vi "GeoData.vi"() -> ()   [LabVIEW 2017] (continued)
TX\tDallas County\tH1\n75007\t48113\tCarrollton\tTX\tDallas County\tH1\n76065\t48113\tMidlothian\tTX\tDallas County\tH1\n75376\t48113\tDallas\tTX\tDallas County\tH1\n75382\t48113\tDallas\tTX\tDallas County\tH1\n75015\t48113\tIrving\tTX\tDallas County\tH1\n75185\t48113\tMesquite\tTX\tDallas County\tH1\n75260\t48113\tDallas\tTX\tDallas County\tH1\n75030\t48113\tRowlett\tTX\tDallas County\tH1\n75125\t48113\tFerris\tTX\tDallas County\tH1\n75206\t48113\tDallas\tTX\tDallas County\tH1\n75229\t48113\tDallas\tTX\tDallas County\tH1\n75218\t48113\tDallas\tTX\tDallas County\tH1\n75248\t48113\tDallas\tTX\tDallas County\tH1\n75054\t48113\tGrand prairie\tTX\tDallas County\tH1\n75082\t48113\tRichardson\tTX\tDallas County\tH1\n75182\t48113\tSunnyvale\tTX\tDallas County\tH1\n75380\t48113\tDallas\tTX\tDallas County\tH1\n75313\t48113\tDallas\tTX\tDallas County\tH1\n75367\t48113\tDallas\tTX\tDallas County\tH1\n75038\t48113\tIrving\tTX\tDallas County\tH1\n75042\t48113\tGarland\tTX\tDallas County\tH1\n75052\t48113\tGrand prairie\tTX\tDallas County\tH1\n75104\t48113\tCedar hill\tTX\tDallas County\tH1\n75150\t48113\tMesquite\tTX\tDallas County\tH1\n75207\t48113\tDallas\tTX\tDallas County\tH1\n75154\t48113\tRed oak\tTX\tDallas County\tH1\n75209\t48113\tDallas\tTX\tDallas County\tH1\n75219\t48113\tDallas\tTX\tDallas County\tH1\n75222\t48113\tDallas\tTX\tDallas County\tH1\n75063\t48113\tIrving\tTX\tDallas County\tH1\n75083\t48113\tRichardson\tTX\tDallas County\tH1\n75081\t48113\tRichardson\tTX\tDallas County\tH1\n75270\t48113\tDallas\tTX\tDallas County\tH1\n75381\t48113\tDallas\tTX\tDallas County\tH1\n75017\t48113\tIrving\tTX\tDallas County\tH1\n75372\t48113\tDallas\tTX\tDallas County\tH1\n79713\t48115\tAckerly\tTX\tDawson County\tH1\n79331\t48115\tLamesa\tTX\tDawson County\tH1\n79377\t48115\tWelch\tTX\tDawson County\tH1\n79351\t48115\tOdonnell\tTX\tDawson County\tH1\n79045\t48117\tHereford\tTX\tDeaf Smith County\tH1\n79098\t48117\tWildorado\tTX\tDeaf Smith County\tH1\n79025\t48117\tDawn\tTX\tDeaf Smith County\tH1\n79092\t48117\tVega\tTX\tDeaf Smith County\tH1\n79035\t48117\tFriona\tTX\tDeaf Smith County\tH1\n79085\t48117\tSummerfield\tTX\tDeaf Smith County\tH1\n79015\t48117\tCanyon\tTX\tDeaf Smith County\tH1\n75469\t48119\tPecan gap\tTX\tDelta County\tH1\n75432\t48119\tCooper\tTX\tDelta County\tH1\n75428\t48119\tCommerce\tTX\tDelta County\tH1\n75450\t48119\tLake creek\tTX\tDelta County\tH1\n75415\t48119\tBen franklin\tTX\tDelta County\tH1\n75448\t48119\tKlondike\tTX\tDelta County\tH1\n75449\t48119\tLadonia\tTX\tDelta County\tH1\n75441\t48119\tEnloe\tTX\tDelta County\tH1\n75067\t48121\tLewisville\tTX\tDenton County\tH1\n76207\t48121\tDenton\tTX\tDenton County\tH1\n76259\t48121\tPonder\tTX\tDenton County\tH1\n76202\t48121\tDenton\tTX\tDenton County\tH1\n76078\t48121\tRhome\tTX\tDenton County\tH1\n76262\t48121\tRoanoke\tTX\tDenton County\tH1\n76258\t48121\tPilot point\tTX\tDenton County\tH1\n75029\t48121\tLewisville\tTX\tDenton County\tH1\n76206\t48121\tDenton\tTX\tDenton County\tH1\n75033\t48121\tFrisco\tTX\tDenton County\tH1\n75077\t48121\tLewisville\tTX\tDenton County\tH1\n75010\t48121\tCarrollton\tTX\tDenton County\tH1\n76205\t48121\tDenton\tTX\tDenton County\tH1\n76210\t48121\tDenton\tTX\tDenton County\tH1\n76177\t48121\tFort worth\tTX\tDenton County\tH1\n76204\t48121\tDenton\tTX\tDenton County\tH1\n75019\t48121\tCoppell\tTX\tDenton County\tH1\n75287\t48121\tDallas\tTX\tDenton County\tH1\n76092\t48121\tSouthlake\tTX\tDenton County\tH1\n76234\t48121\tDecatur\tTX\tDenton County\tH1\n76247\t48121\tJustin\tTX\tDenton County\tH1\n75065\t48121\tLake dallas\tTX\tDenton County\tH1\n75009\t48121\tCelina\tTX\tDenton County\tH1\n76208\t48121\tDenton\tTX\tDenton County\tH1\n76226\t48121\tArgyle\tTX\tDenton County\tH1\n75011\t48121\tCarrollton\tTX\tDenton County\tH1\n75028\t48121\tFlower mound\tTX\tDenton County\tH1\n75093\t48121\tPlano\tTX\tDenton County\tH1\n75007\t48121\tCarrollton\tTX\tDenton County\tH1\n76249\t48121\tKrum\tTX\tDenton County\tH1\n76201\t48121\tDenton\tTX\tDenton County\tH1\n76266\t48121\tSanger\tTX\tDenton County\tH1\n75027\t48121\tFlower mound\tTX\tDenton County\tH1\n75022\t48121\tFlower mound\tTX\tDenton County\tH1\n75024\t48121\tPlano\tTX\tDenton County\tH1\n75057\t48121\tLewisville\tTX\tDenton County\tH1\n76052\t48121\tHaslet\tTX\tDenton County\tH1\n76209\t48121\tDenton\tTX\tDenton County\tH1\n76203\t48121\tDenton\tTX\tDenton County\tH1\n75034\t48121\tFrisco\tTX\tDenton County\tH1\n75035\t48121\tFrisco\tTX\tDenton County\tH1\n75068\t48121\tLittle elm\tTX\tDenton County\tH1\n75056\t48121\tThe colony\tTX\tDenton County\tH1\n75078\t48121\tProsper\tTX\tDenton County\tH1\n76227\t48121\tAubrey\tTX\tDenton County\tH1\n76272\t48121\tValley view\tTX\tDenton County\tH1\n77967\t48123\tHochheim\tTX\tDeWitt County\tH1\n77954\t48123\tCuero\tTX\tDeWitt County\tH1\n77984\t48123\tShiner\tTX\tDeWitt County\tH1\n77974\t48123\tMeyersville\tTX\tDeWitt County\tH1\n78141\t48123\tNordheim\tTX\tDeWitt County\tH1\n77989\t48123\tThomaston\tTX\tDeWitt County\tH1\n77995\t48123\tYoakum\tTX\tDeWitt County\tH1\n77994\t48123\tWesthoff\tTX\tDeWitt County\tH1\n78164\t48123\tYorktown\tTX\tDeWitt County\tH1\n79256\t48125\tRoaring springs\tTX\tDickens County\tH1\n79370\t48125\tSpur\tTX\tDickens County\tH1\n79220\t48125\tAfton\tTX\tDickens County\tH1\n79229\t48125\tDickens\tTX\tDickens County\tH1\n79243\t48125\tMcadoo\tTX\tDickens County\tH1\n78827\t48127\tAsherton\tTX\tDimmit County\tH1\n78836\t48127\tCatarina\tTX\tDimmit County\tH1\n78834\t48127\tCarrizo springs\tTX\tDimmit County\tH1\n78839\t48127\tCrystal city\tTX\tDimmit County\tH1\n78830\t48127\tBig wells\tTX\tDimmit County\tH1\n79065\t48129\tPampa\tTX\tDonley County\tH1\n79237\t48129\tHedley\tTX\tDonley County\tH1\n79057\t48129\tMclean\tTX\tDonley County\tH1\n79226\t48129\tClarendon\tTX\tDonley County\tH1\n79240\t48129\tLelia lake\tTX\tDonley County\tH1\n78357\t48131\tFreer\tTX\tDuval County\tH1\n78384\t48131\tSan diego\tTX\tDuval County\tH1\n78332\t48131\tAlice\tTX\tDuval County\tH1\n78349\t48131\tConcepcion\tTX\tDuval County\tH1\n78376\t48131\tRealitos\tTX\tDuval County\tH1\n78341\t48131\tBenavides\tTX\tDuval County\tH1\n76435\t48133\tCarbon\tTX\tEastland County\tH1\n76470\t48133\tRanger\tTX\tEastland County\tH1\n76471\t48133\tRising star\tTX\tEastland County\tH1\n76466\t48133\tOlden\tTX\tEastland County\tH1\n76442\t48133\tComanche\tTX\tEastland County\tH1\n76444\t48133\tDe leon\tTX\tEastland County\tH1\n76437\t48133\tCisco\tTX\tEastland County\tH1\n76464\t48133\tMoran\tTX\tEastland County\tH1\n76445\t48133\tDesdemona\tTX\tEastland County\tH1\n76443\t48133\tCross plains\tTX\tEastland County\tH1\n76448\t48133\tEastland\tTX\tEastland County\tH1\n76454\t48133\tGorman\tTX\tEastland County\tH1\n79760\t48135\tOdessa\tTX\tEctor County\tH1\n79762\t48135\tOdessa\tTX\tEctor County\tH1\n79707\t48135\tMidland\tTX\tEctor County\tH1\n79763\t48135\tOdessa\tTX\tEctor County\tH1\n79765\t48135\tOdessa\tTX\tEctor County\tH1\n79768\t48135\tOdessa\tTX\tEctor County\tH1\n79741\t48135\tGoldsmith\tTX\tEctor County\tH1\n79761\t48135\tOdessa\tTX\tEctor County\tH1\n79764\t48135\tOdessa\tTX\tEctor County\tH1\n79758\t48135\tGardendale\tTX\tEctor County\tH1\n79766\t48135\tOdessa\tTX\tEctor County\tH1\n79776\t48135\tPenwell\tTX\tEctor County\tH1\n79769\t48135\tOdessa\tTX\tEctor County\tH1\n79759\t48135\tNotrees\tTX\tEctor County\tH1\n78833\t48137\tCamp wood\tTX\tEdwards County\tH1\n78880\t48137\tRocksprings\tTX\tEdwards County\tH1\n78840\t48137\tDel rio\tTX\tEdwards County\tH1\n78828\t48137\tBarksdale\tTX\tEdwards County\tH1\n75146\t48139\tLancaster\tTX\tEllis County\tH1\n76055\t48139\tItasca\tTX\tEllis County\tH1\n75152\t48139\tPalmer\tTX\tEllis County\tH1\n76084\t48139\tVenus\tTX\tEllis County\tH1\n76041\t48139\tForreston\tTX\tEllis County\tH1\n75165\t48139\tWaxahachie\tTX\tEllis County\tH1\n76641\t48139\tFrost\tTX\tEllis County\tH1\n76651\t48139\tItaly\tTX\tEllis County\tH1\n76626\t48139\tBlooming grove\tTX\tEllis County\tH1\n75119\t48139\tEnnis\tTX\tEllis County\tH1\n75167\t48139\tWaxahachie\tTX\tEllis County\tH1\n76050\t48139\tGrandview\tTX\tEllis County\tH1\n76064\t48139\tMaypearl\tTX\tEllis County\tH1\n76065\t48139\tMidlothian\tTX\tEllis County\tH1\n75168\t48139\tWaxahachie\tTX\tEllis County\tH1\n75125\t48139\tFerris\tTX\tEllis County\tH1\n76063\t48139\tMansfield\tTX\tEllis County\tH1\n76670\t48139\tMilford\tTX\tEllis County\tH1\n75104\t48139\tCedar hill\tTX\tEllis County\tH1\n75154\t48139\tRed oak\tTX\tEllis County\tH1\n76623\t48139\tAvalon\tTX\tEllis County\tH1\n75101\t48139\tBardwell\tTX\tEllis County\tH1\n79836\t48141\tClint\tTX\tEl Paso County\tH1\n79923\t48141\tEl paso\tTX\tEl Paso County\tH1\n79932\t48141\tEl paso\tTX\tEl Paso County\tH1\n79936\t48141\tEl paso\tTX\tEl Paso County\tH1\n79931\t48141\tEl paso\tTX\tEl Paso County\tH1\n79948\t48141\tEl paso\tTX\tEl Paso County\tH1\n79953\t48141\tEl paso\tTX\tEl Paso County\tH1\n79905\t48141\tEl paso\tTX\tEl Paso County\tH1\n79914\t48141\tEl paso\tTX\tEl Paso County\tH1\n79927\t48141\tEl paso\tTX\tEl Paso County\tH1\n79911\t48141\tEl paso\tTX\tEl Paso County\tH1\n79937\t48141\tEl paso\tTX\tEl Paso County\tH1\n79910\t48141\tEl paso\tTX\tEl Paso County\tH1\n79912\t48141\tEl paso\tTX\tEl Paso County\tH1\n79915\t48141\tEl paso\tTX\tEl Paso County\tH1\n79930\t48141\tEl paso\tTX\tEl Paso County\tH1\n79926\t48141\tEl paso\tTX\tEl Paso County\tH1\n79944\t48141\tEl paso\tTX\tEl Paso County\tH1\n79935\t48141\tEl paso\tTX\tEl Paso County\tH1\n79996\t48141\tEl paso\tTX\tEl Paso County\tH1\n79942\t48141\tEl paso\tTX\tEl Paso County\tH1\n79968\t48141\tEl paso\tTX\tEl Paso County\tH1\n79954\t48141\tEl paso\tTX\tEl Paso County\tH1\n79835\t48141\tCanutillo\tTX\tEl Paso County\tH1\n79902\t48141\tEl paso\tTX\tEl Paso County\tH1\n79907\t48141\tEl paso\tTX\tEl Paso County\tH1\n79849\t48141\tSan elizario\tTX\tEl Paso County\tH1\n79903\t48141\tEl paso\tTX\tEl Paso County\tH1\n79908\t48141\tEl paso\tTX\tEl Paso County\tH1\n79941\t48141\tEl paso\tTX\tEl Paso County\tH1\n79951\t48141\tEl paso\tTX\tEl Paso County\tH1\n79952\t48141\tEl paso\tTX\tEl Paso County\tH1\n79940\t48141\tEl paso\tTX\tEl Paso County\tH1\n79924\t48141\tEl paso\tTX\tEl Paso County\tH1\n79904\t48141\tEl paso\tTX\tEl Paso County\tH1\n79906\t48141\tEl paso\tTX\tEl Paso County\tH1\n79938\t48141\tEl paso\tTX\tEl Paso County\tH1\n79934\t48141\tEl paso\tTX\tEl Paso County\tH1\n79821\t48141\tAnthony\tTX\tEl Paso County\tH1\n79913\t48141\tEl paso\tTX\tEl Paso County\tH1\n79955\t48141\tEl paso\tTX\tEl Paso County\tH1\n79838\t48141\tFabens\tTX\tEl Paso County\tH1\n79946\t48141\tEl paso\tTX\tEl Paso County\tH1\n79901\t48141\tEl paso\tTX\tEl Paso County\tH1\n79922\t48141\tEl paso\tTX\tEl Paso County\tH1\n79928\t48141\tEl paso\tTX\tEl Paso County\tH1\n79997\t48141\tEl paso\tTX\tEl Paso County\tH1\n79950\t48141\tEl paso\tTX\tEl Paso County\tH1\n79995\t48141\tEl paso\tTX\tEl Paso County\tH1\n79945\t48141\tEl paso\tTX\tEl Paso County\tH1\n79918\t48141\tFort bliss\tTX\tEl Paso County\tH1\n79925\t48141\tEl paso\tTX\tEl Paso County\tH1\n79943\t48141\tEl paso\tTX\tEl Paso County\tH1\n79917\t48141\tEl paso\tTX\tEl Paso County\tH1\n79916\t48141\tFort bliss\tTX\tEl Paso County\tH1\n79929\t48141\tEl paso\tTX\tEl Paso County\tH1\n79947\t48141\tEl paso\tTX\tEl Paso County\tH1\n79853\t48141\tTornillo\tTX\tEl Paso County\tH1\n79949\t48141\tEl paso\tTX\tEl Paso County\tH1\n76436\t48143\tCarlton\tTX\tErath County\tH1\n76462\t48143\tLipan\tTX\tErath County\tH1\n76401\t48143\tStephenville\tTX\tErath County\tH1\n76453\t48143\tGordon\tTX\tErath County\tH1\n76461\t48143\tLingleville\tTX\tErath County\tH1\n76446\t48143\tDublin\tTX\tErath County\tH1\n76457\t48143\tHico\tTX\tErath County\tH1\n76433\t48143\tBluff dale\tTX\tErath County\tH1\n76649\t48143\tIredell\tTX\tErath County\tH1\n76465\t48143\tMorgan mill\tTX\tErath County\tH1\n76444\t48143\tDe leon\tTX\tErath County\tH1\n76445\t48143\tDesdemona\tTX\tErath County\tH1\n76463\t48143\tMingus\tTX\tErath County\tH1\n76402\t48143\tStephenville\tTX\tErath County\tH1\n76629\t48145\tBremond\tTX\tFalls County\tH1\n76664\t48145\tMart\tTX\tFalls County\tH1\n76519\t48145\tBurlington\tTX\tFalls County\tH1\n76579\t48145\tTroy\tTX\tFalls County\tH1\n76655\t48145\tLorena\tTX\tFalls County\tH1\n76632\t48145\tChilton\tTX\tFalls County\tH1\n76630\t48145\tBruceville\tTX\tFalls County\tH1\n76682\t48145\tRiesel\tTX\tFalls County\tH1\n76570\t48145\tRosebud\tTX\tFalls County\tH1\n76706\t48145\tWaco\tTX\tFalls County\tH1\n76653\t48145\tKosse\tTX\tFalls County\tH1\n76680\t48145\tReagan\tTX\tFalls County\tH1\n76524\t48145\tEddy\tTX\tFalls County\tH1\n76661\t48145\tMarlin\tTX\tFalls County\tH1\n76685\t48145\tSatin\tTX\tFalls County\tH1\n76656\t48145\tLott\tTX\tFalls County\tH1\n75414\t48147\tBells\tTX\tFannin County\tH1\n75469\t48147\tPecan gap\tTX\tFannin County\tH1\n75438\t48147\tDodd city\tTX\tFannin County\tH1\n75423\t48147\tCeleste\tTX\tFannin County\tH1\n75447\t48147\tIvanhoe\tTX\tFannin County\tH1\n75418\t48147\tBonham\tTX\tFannin County\tH1\n75479\t48147\tSavoy\tTX\tFannin County\tH1\n75439\t48147\tEctor\tTX\tFannin County\tH1\n75476\t48147\tRavenna\tTX\tFannin County\tH1\n75475\t48147\tRandolph\tTX\tFannin County\tH1\n75496\t48147\tWolfe city\tTX\tFannin County\tH1\n75443\t48147\tGober\tTX\tFannin County\tH1\n75452\t48147\tLeonard\tTX\tFannin County\tH1\n75490\t48147\tTrenton\tTX\tFannin County\tH1\n75488\t48147\tTelephone\tTX\tFannin County\tH1\n75449\t48147\tLadonia\tTX\tFannin County\tH1\n75413\t48147\tBailey\tTX\tFannin County\tH1\n75424\t48147\tBlue ridge\tTX\tFannin County\tH1\n75446\t48147\tHoney grove\tTX\tFannin County\tH1\n75491\t48147\tWhitewright\tTX\tFannin County\tH1\n75492\t48147\tWindom\tTX\tFannin County\tH1\n78942\t48149\tGiddings\tTX\tFayette County\tH1\n78932\t48149\tCarmine\tTX\tFayette County\tH1\n78934\t48149\tColumbus\tTX\tFayette County\tH1\n78959\t48149\tWaelder\tTX\tFayette County\tH1\n78952\t48149\tPlum\tTX\tFayette County\tH1\n78949\t48149\tMuldoon\tTX\tFayette County\tH1\n78951\t48149\tOakland\tTX\tFayette County\tH1\n78941\t48149\tFlatonia\tTX\tFayette County\tH1\n78940\t48149\tFayetteville\tTX\tFayette County\tH1\n78956\t48149\tSchulenburg\tTX\tFayette County\tH1\n78946\t48149\tLedbetter\tTX\tFayette County\tH1\n78935\t48149\tAlleyton\tTX\tFayette County\tH1\n78954\t48149\tRound top\tTX\tFayette County\tH1\n78957\t48149\tSmithville\tTX\tFayette County\tH1\n78962\t48149\tWeimar\tTX\tFayette County\tH1\n78961\t48149\tWarrenton\tTX\tFayette County\tH1\n78960\t48149\tWarda\tTX\tFayette County\tH1\n78963\t48149\tWest point\tTX\tFayette County\tH1\n78950\t48149\tNew ulm\tTX\tFayette County\tH1\n78938\t48149\tEllinger\tTX\tFayette County\tH1\n78945\t48149\tLa grange\tTX\tFayette County\tH1\n79526\t48151\tHermleigh\tTX\tFisher County\tH1\n79520\t48151\tHamlin\tTX\tFisher County\tH1\n79545\t48151\tRoscoe\tTX\tFisher County\tH1\n79534\t48151\tMc caulley\tTX\tFisher County\tH1\n79543\t48151\tRoby\tTX\tFisher County\tH1\n79546\t48151\tRotan\tTX\tFisher County\tH1\n79560\t48151\tSylvester\tTX\tFisher County\tH1\n79556\t48151\tSweetwater\tTX\tFisher County\tH1\n79231\t48153\tDougherty\tTX\tFloyd County\tH1\n79241\t48153\tLockney\tTX\tFloyd County\tH1\n79235\t48153\tFloydada\tTX\tFloyd County\tH1\n79258\t48153\tSouth plains\tTX\tFloyd County\tH1\n79221\t48153\tAiken\tTX\tFloyd County\tH1\n79227\t48155\tCrowell\tTX\tFoard County\tH1\n76384\t48155\tVernon\tTX\tFoard County\tH1\n79248\t48155\tPaducah\tTX\tFoard County\tH1\n77469\t48157\tRichmond\tTX\tFort Bend County\tH1\n77489\t48157\tMissouri city\tTX\tFort Bend County\tH1\n77584\t48157\tPearland\tTX\tFort Bend County\tH1\n77476\t48157\tSimonton\tTX\tFort Bend County\tH1\n77417\t48157\tBeasley\tTX\tFort Bend County\tH1\n77031\t48157\tHouston\tTX\tFort Bend County\tH1\n77461\t48157\tNeedville\tTX\tFort Bend County\tH1\n77082\t48157\tHouston\tTX\tFort Bend County\tH1\n77407\t48157\tRichmond\tTX\tFort Bend County\tH1\n77441\t48157\tFulshear\tTX\tFort Bend County\tH1\n77471\t48157\tRosenberg\tTX\tFort Bend County\tH1\n77493\t48157\tKaty\tTX\tFort Bend County\tH1\n77487\t48157\tSugar land\tTX\tFort Bend County\tH1\n77497\t48157\tStafford\tTX\tFort Bend County\tH1\n77085\t48157\tHouston\tTX\tFort Bend County\tH1\n77423\t48157\tBrookshire\tTX\tFort Bend County\tH1\n77435\t48157\tEast bernard\tTX\tFort Bend County\tH1\n77420\t48157\tBoling\tTX\tFort Bend County\tH1\n77478\t48157\tSugar land\tTX\tFort Bend County\tH1\n77496\t48157\tSugar land\tTX\tFort Bend County\tH1\n77451\t48157\tKendleton\tTX\tFort Bend County\tH1\n77406\t48157\tRichmond\tTX\tFort Bend County\tH1\n77450\t48157\tKaty\tTX\tFort Bend County\tH1\n77498\t48157\tSugar land\tTX\tFort Bend County\tH1\n77583\t48157\tRosharon\tTX\tFort Bend County\tH1\n77464\t48157\tOrchard\tTX\tFort Bend County\tH1\n77430\t48157\tDamon\tTX\tFort Bend County\tH1\n77459\t48157\tMissouri city\tTX\tFort Bend County\tH1\n77444\t48157\tGuy\tTX\tFort Bend County\tH1\n77083\t48157\tHouston\tTX\tFort Bend County\tH1\n77053\t48157\tHouston\tTX\tFort Bend County\tH1\n77479\t48157\tSugar land\tTX\tFort Bend County\tH1\n77545\t48157\tFresno\tTX\tFort Bend County\tH1\n77481\t48157\tThompsons\tTX\tFort Bend County\tH1\n77099\t48157\tHouston\tTX\tFort Bend County\tH1\n77485\t48157\tWallis\tTX\tFort Bend County\tH1\n77494\t48157\tKaty\tTX\tFort Bend County\tH1\n77477\t48157\tStafford\tTX\tFort Bend County\tH1\n75457\t48159\tMount vernon\tTX\tFranklin County\tH1\n75480\t48159\tScroggins\tTX\tFranklin County\tH1\n75455\t48159\tMount pleasant\tTX\tFranklin County\tH1\n75481\t48159\tSulphur bluff\tTX\tFranklin County\tH1\n75494\t48159\tWinnsboro\tTX\tFranklin County\tH1\n75487\t48159\tTalco\tTX\tFranklin County\tH1\n75478\t48159\tSaltillo\tTX\tFranklin County\tH1\n75838\t48161\tDonie\tTX\tFreestone County\tH1\n75859\t48161\tStreetman\tTX\tFreestone County\tH1\n75840\t48161\tFairfield\tTX\tFreestone County\tH1\n76667\t48161\tMexia\tTX\tFreestone County\tH1\n75831\t48161\tBuffalo\tTX\tFreestone County\tH1\n75855\t48161\tOakwood\tTX\tFreestone County\tH1\n76693\t48161\tWortham\tTX\tFreestone County\tH1\n75848\t48161\tKirvin\tTX\tFreestone County\tH1\n75860\t48161\tTeague\tTX\tFreestone County\tH1\n78017\t48163\tDilley\tTX\tFrio County\tH1\n78061\t48163\tPearsall\tTX\tFrio County\tH1\n78016\t48163\tDevine\tTX\tFrio County\tH1\n78057\t48163\tMoore\tTX\tFrio County\tH1\n78005\t48163\tBigfoot\tTX\tFrio County\tH1\n79359\t48165\tSeagraves\tTX\tGaines County\tH1\n79360\t48165\tSeminole\tTX\tGaines County\tH1\n79323\t48165\tDenver city\tTX\tGaines County\tH1\n79342\t48165\tLoop\tTX\tGaines County\tH1\n77510\t48167\tSanta fe\tTX\tGalveston County\tH1\n77553\t48167\tGalveston\tTX\tGalveston County\tH1\n77650\t48167\tPort bolivar\tTX\tGalveston County\tH1\n77555\t48167\tGalveston\tTX\tGalveston County\tH1\n77539\t48167\tDickinson\tTX\tGalveston County\tH1\n77552\t48167\tGalveston\tTX\tGalveston County\tH1\n77517\t48167\tSanta fe\tTX\tGalveston County\tH1\n77546\t48167\tFriendswood\tTX\tGalveston County\tH1\n77554\t48167\tGalveston\tTX\tGalveston County\tH1\n77549\t48167\tFriendswood\tTX\tGalveston County\tH1\n77565\t48167\tKemah\tTX\tGalveston County\tH1\n77581\t48167\tPearland\tTX\tGalveston County\tH1\n77623\t48167\tHigh island\tTX\tGalveston County\tH1\n77551\t48167\tGalveston\tTX\tGalveston County\tH1\n77563\t48167\tHitchcock\tTX\tGalveston County\tH1\n77591\t48167\tTexas city\tTX\tGalveston County\tH1\n77573\t48167\tLeague city\tTX\tGalveston County\tH1\n77568\t48167\tLa marque\tTX\tGalveston County\tH1\n77574\t48167\tLeague city\tTX\tGalveston County\tH1\n77511\t48167\tAlvin\tTX\tGalveston County\tH1\n77550\t48167\tGalveston\tTX\tGalveston County\tH1\n77518\t48167\tBacliff\tTX\tGalveston County\tH1\n77590\t48167\tTexas city\tTX\tGalveston County\tH1\n79356\t48169\tPost\tTX\tGarza County\tH1\n79330\t48169\tJusticeburg\tTX\tGarza County\tH1\n78624\t48171\tFredericksburg\tTX\tGillespie County\tH1\n76856\t48171\tMason\tTX\tGillespie County\tH1\n78631\t48171\tHarper\tTX\tGillespie County\tH1\n78058\t48171\tMountain home\tTX\tGillespie County\tH1\n78028\t48171\tKerrville\tTX\tGillespie County\tH1\n78675\t48171\tWillow city\tTX\tGillespie County\tH1\n78671\t48171\tStonewall\tTX\tGillespie County\tH1\n78618\t48171\tDoss\tTX\tGillespie County\tH1\n79720\t48173\tBig spring\tTX\tGlasscock County\tH1\n79739\t48173\tGarden city\tTX\tGlasscock County\tH1\n77960\t48175\tFannin\tTX\tGoliad County\tH1\n78119\t48175\tKenedy\tTX\tGoliad County\tH1\n77963\t48175\tGoliad\tTX\tGoliad County\tH1\n78107\t48175\tBerclair\tTX\tGoliad County\tH1\n77905\t48175\tVictoria\tTX\tGoliad County\tH1\n77993\t48175\tWeesatche\tTX\tGoliad County\tH1\n78164\t48175\tYorktown\tTX\tGoliad County\tH1\n78959\t48177\tWaelder\tTX\tGonzales County\tH1\n78632\t48177\tHarwood\tTX\tGonzales County\tH1\n78941\t48177\tFlatonia\tTX\tGonzales County\tH1\n77984\t48177\tShiner\tTX\tGonzales County\tH1\n78629\t48177\tGonzales\tTX\tGonzales County\tH1\n78122\t48177\tLeesville\tTX\tGonzales County\tH1\n78614\t48177\tCost\tTX\tGonzales County\tH1\n78677\t48177\tWrightsboro\tTX\tGonzales County\tH1\n78159\t48177\tSmiley\tTX\tGonzales County\tH1\n78648\t48177\tLuling\tTX\tGonzales County\tH1\n77994\t48177\tWesthoff\tTX\tGonzales County\tH1\n78140\t48177\tNixon\tTX\tGonzales County\tH1\n78604\t48177\tBelmont\tTX\tGonzales County\tH1\n79079\t48179\tShamrock\tTX\tGray County\tH1\n79065\t48179\tPampa\tTX\tGray County\tH1\n79066\t48179\tPampa\tTX\tGray County\tH1\n79057\t48179\tMclean\tTX\tGray County\tH1\n79054\t48179\tLefors\tTX\tGray County\tH1\n79097\t48179\tWhite deer\tTX\tGray County\tH1\n79039\t48179\tGroom\tTX\tGray County\tH1\n79061\t48179\tMobeetie\tTX\tGray County\tH1\n79002\t48179\tAlanreed\tTX\tGray County\tH1\n75021\t48181\tDenison\tTX\tGrayson County\tH1\n75414\t48181\tBells\tTX\tGrayson County\tH1\n75092\t48181\tSherman\tTX\tGrayson County\tH1\n75058\t48181\tGunter\tTX\tGrayson County\tH1\n75459\t48181\tHowe\tTX\tGrayson County\tH1\n76258\t48181\tPilot point\tTX\tGrayson County\tH1\n75479\t48181\tSavoy\tTX\tGrayson County\tH1\n76233\t48181\tCollinsville\tTX\tGrayson County\tH1\n76240\t48181\tGainesville\tTX\tGrayson County\tH1\n76271\t48181\tTioga\tTX\tGrayson County\tH1\n76268\t48181\tSouthmayd\tTX\tGrayson County\tH1\n75020\t48181\tDenison\tTX\tGrayson County\tH1\n75009\t48181\tCelina\tTX\tGrayson County\tH1\n75090\t48181\tSherman\tTX\tGrayson County\tH1\n75076\t48181\tPottsboro\tTX\tGrayson County\tH1\n75490\t48181\tTrenton\tTX\tGrayson County\tH1\n76273\t48181\tWhitesboro\tTX\tGrayson County\tH1\n75091\t48181\tSherman\tTX\tGrayson County\tH1\n76264\t48181\tSadler\tTX\tGrayson County\tH1\n75495\t48181\tVan alstyne\tTX\tGrayson County\tH1\n75489\t48181\tTom bean\tTX\tGrayson County\tH1\n75491\t48181\tWhitewright\tTX\tGrayson County\tH1\n76245\t48181\tGordonville\tTX\tGrayson County\tH1\n75605\t48183\tLongview\tTX\tGregg County\tH1\n75607\t48183\tLongview\tTX\tGregg County\tH1\n75604\t48183\tLongview\tTX\tGregg County\tH1\n75663\t48183\tKilgore\tTX\tGregg County\tH1\n75601\t48183\tLongview\tTX\tGregg County\tH1\n75602\t48183\tLongview\tTX\tGregg County\tH1\n75691\t48183\tTatum\tTX\tGregg County\tH1\n75608\t48183\tLongview\tTX\tGregg County\tH1\n75606\t48183\tLongview\tTX\tGregg County\tH1\n75615\t48183\tLongview\tTX\tGregg County\tH1\n75603\t48183\tLongview\tTX\tGregg County\tH1\n75641\t48183\tEaston\tTX\tGregg County\tH1\n75660\t48183\tJudson\tTX\tGregg County\tH1\n75645\t48183\tGilmer\tTX\tGregg County\tH1\n75647\t48183\tGladewater\tTX\tGregg County\tH1\n75662\t48183\tKilgore\tTX\tGregg County\tH1\n75693\t48183\tWhite oak\tTX\tGregg County\tH1\n77356\t48185\tMontgomery\tTX\tGrimes County\tH1\n77868\t48185\tNavasota\tTX\tGrimes County\tH1\n77875\t48185\tRoans prairie\tTX\tGrimes County\tH1\n77872\t48185\tNorth zulch\tTX\tGrimes County\tH1\n77861\t48185\tIola\tTX\tGrimes County\tH1\n77830\t48185\tAnderson\tTX\tGrimes County\tH1\n77873\t48185\tRichards\tTX\tGrimes County\tH1\n77831\t48185\tBedias\tTX\tGrimes County\tH1\n77316\t48185\tMontgomery\tTX\tGrimes County\tH1\n77363\t48185\tPlantersville\tTX\tGrimes County\tH1\n77484\t48185\tWaller\tTX\tGrimes County\tH1\n77876\t48185\tShiro\tTX\tGrimes County\tH1\n78132\t48187\tNew braunfels\tTX\tGuadalupe County\tH1\n78124\t48187\tMarion\tTX\tGuadalupe County\tH1\n78115\t48187\tGeronimo\tTX\tGuadalupe County\tH1\n78130\t48187\tNew braunfels\tTX\tGuadalupe County\tH1\n78156\t48187\tSeguin\tTX\tGuadalupe County\tH1\n78108\t48187\tCibolo\tTX\tGuadalupe County\tH1\n78155\t48187\tSeguin\tTX\tGuadalupe County\tH1\n78666\t48187\tSan marcos\tTX\tGuadalupe County\tH1\n78123\t48187\tMc queeney\tTX\tGuadalupe County\tH1\n78154\t48187\tSchertz\tTX\tGuadalupe County\tH1\n78648\t48187\tLuling\tTX\tGuadalupe County\tH1\n78638\t48187\tKingsbury\tTX\tGuadalupe County\tH1\n78670\t48187\tStaples\tTX\tGuadalupe County\tH1\n78121\t48187\tLa vernia\tTX\tGuadalupe County\tH1\n78140\t48187\tNixon\tTX\tGuadalupe County\tH1\n78655\t48187\tMartindale\tTX\tGuadalupe County\tH1\n79064\t48189\tOlton\tTX\tHale County\tH1\n79021\t48189\tCotton center\tTX\tHale County\tH1\n79073\t48189\tPlainview\tTX\tHale County\tH1\n79032\t48189\tEdmonson\tTX\tHale County\tH1\n79072\t48189\tPlainview\tTX\tHale County\tH1\n79041\t48189\tHale center\tTX\tHale County\tH1\n79311\t48189\tAbernathy\tTX\tHale County\tH1\n79250\t48189\tPetersburg\tTX\tHale County\tH1\n79261\t48191\tTurkey\tTX\tHall County\tH1\n79233\t48191\tEstelline\tTX\tHall County\tH1\n79226\t48191\tClarendon\tTX\tHall County\tH1\n79255\t48191\tQuitaque\tTX\tHall County\tH1\n79239\t48191\tLakeview\tTX\tHall County\tH1\n79201\t48191\tChildress\tTX\tHall County\tH1\n79245\t48191\tMemphis\tTX\tHall County\tH1\n79234\t48191\tFlomot\tTX\tHall County\tH1\n79259\t48191\tTell\tTX\tHall County\tH1\n76436\t48193\tCarlton\tTX\tHamilton County\tH1\n76531\t48193\tHamilton\tTX\tHamilton County\tH1\n76446\t48193\tDublin\tTX\tHamilton County\tH1\n76457\t48193\tHico\tTX\tHamilton County\tH1\n76649\t48193\tIredell\tTX\tHamilton County\tH1\n76844\t48193\tGoldthwaite\tTX\tHamilton County\tH1\n76538\t48193\tJonesboro\tTX\tHamilton County\tH1\n76565\t48193\tPottsville\tTX\tHamilton County\tH1\n76525\t48193\tEvant\tTX\tHamilton County\tH1\n76637\t48193\tCranfills gap\tTX\tHamilton County\tH1\n79062\t48195\tMorse\tTX\tHansford County\tH1\n79081\t48195\tSpearman\tTX\tHansford County\tH1\n79083\t48195\tStinnett\tTX\tHansford County\tH1\n79040\t48195\tGruver\tTX\tHansford County\tH1\n79247\t48197\tOdell\tTX\tHardeman County\tH1\n79252\t48197\tQuanah\tTX\tHardeman County\tH1\n79225\t48197\tChillicothe\tTX\tHardeman County\tH1\n77585\t48199\tSaratoga\tTX\tHardin County\tH1\n77663\t48199\tVillage mills\tTX\tHardin County\tH1\n77374\t48199\tThicket\tTX\tHardin County\tH1\n77705\t48199\tBeaumont\tTX\tHardin County\tH1\n77625\t48199\tKountze\tTX\tHardin County\tH1\n77564\t48199\tHull\tTX\tHardin County\tH1\n77376\t48199\tVotaw\tTX\tHardin County\tH1\n77659\t48199\tSour lake\tTX\tHardin County\tH1\n77657\t48199\tLumberton\tTX\tHardin County\tH1\n77664\t48199\tWarren\tTX\tHardin County\tH1\n77519\t48199\tBatson\tTX\tHardin County\tH1\n77656\t48199\tSilsbee\tTX\tHardin County\tH1\n77007\t48201\tHouston\tTX\tHarris County\tH1\n77027\t48201\tHouston\tTX\tHarris County\tH1\n77021\t48201\tHouston\tTX\tHarris County\tH1\n77088\t48201\tHouston\tTX\tHarris County\tH1\n77090\t48201\tHouston\tTX\tHarris County\tH1\n77095\t48201\tHouston\tTX\tHarris County\tH1\n77096\t48201\tHouston\tTX\tHarris County\tH1\n77204\t48201\tHouston\tTX\tHarris County\tH1\n77068\t48201\tHouston\tTX\tHarris County\tH1\n77233\t48201\tHouston\tTX\tHarris County\tH1\n77401\t48201\tBellaire\tTX\tHarris County\tH1\n77042\t48201\tHouston\tTX\tHarris County\tH1\n77044\t48201\tHouston\tTX\tHarris County\tH1\n77054\t48201\tHouston\tTX\tHarris County\tH1\n77035\t48201\tHouston\tTX\tHarris County\tH1\n77037\t48201\tHouston\tTX\tHarris County\tH1\n77065\t48201\tHouston\tTX\tHarris County\tH1\n77060\t48201\tHouston\tTX\tHarris County\tH1\n77489\t48201\tMissouri city\tTX\tHarris County\tH1\n77504\t48201\tPasadena\tTX\tHarris County\tH1\n77506\t48201\tPasadena\tTX\tHarris County\tH1\n77520\t48201\tBaytown\tTX\tHarris County\tH1\n77241\t48201\tHouston\tTX\tHarris County\tH1\n77265\t48201\tHouston\tTX\tHarris County\tH1\n77270\t48201\tHouston\tTX\tHarris County\tH1\n77242\t48201\tHouston\tTX\tHarris County\tH1\n77252\t48201\tHouston\tTX\tHarris County\tH1\n77226\t48201\tHouston\tTX\tHarris County\tH1\n77273\t48201\tHouston\tTX\tHarris County\tH1\n77279\t48201\tHouston\tTX\tHarris County\tH1\n77245\t48201\tHouston\tTX\tHarris County\tH1\n77210\t48201\tHouston\tTX\tHarris County\tH1\n77017\t48201\tHouston\tTX\tHarris County\tH1\n77008\t48201\tHouston\tTX\tHarris County\tH1\n77024\t48201\tHouston\tTX\tHarris County\tH1\n77087\t48201\tHouston\tTX\tHarris County\tH1\n77075\t48201\tHouston\tTX\tHarris County\tH1\n77080\t48201\tHouston\tTX\tHarris County\tH1\n77073\t48201\tHouston\tTX\tHarris County\tH1\n77093\t48201\tHouston\tTX\tHarris County\tH1\n77079\t48201\tHouston\tTX\tHarris County\tH1\n77076\t48201\tHouston\tTX\tHarris County\tH1\n77347\t48201\tHumble\tTX\tHarris County\tH1\n77231\t48201\tHouston\tTX\tHarris County\tH1\n77389\t48201\tSpring\tTX\tHarris County\tH1\n77375\t48201\tTomball\tTX\tHarris County\tH1\n77031\t48201\tHouston\tTX\tHarris County\tH1\n77449\t48201\tKaty\tTX\tHarris County\tH1\n77521\t48201\tBaytown\tTX\tHarris County\tH1\n77546\t48201\tFriendswood\tTX\tHarris County\tH1\n77243\t48201\tHouston\tTX\tHarris County\tH1\n77284\t48201\tHouston\tTX\tHarris County\tH1\n77046\t48201\tHouston\tTX\tHarris County\tH1\n77206\t48201\tHouston\tTX\tHarris County\tH1\n77491\t48201\tKaty\tTX\tHarris County\tH1\n77266\t48201\tHouston\tTX\tHarris County\tH1\n77261\t48201\tHouston\tTX\tHarris County\tH1\n77325\t48201\tKingwood\tTX\tHarris County\tH1\n77230\t48201\tHouston\tTX\tHarris County\tH1\n77253\t48201\tHouston\tTX\tHarris County\tH1\n77201\t48201\tHouston\tTX\tHarris County\tH1\n77015\t48201\tHouston\tTX\tHarris County\tH1\n77012\t48201\tHouston\tTX\tHarris County\tH1\n77013\t48201\tHouston\tTX\tHarris County\tH1\n77082\t48201\tHouston\tTX\tHarris County\tH1\n77071\t48201\tHouston\tTX\tHarris County\tH1\n77074\t48201\tHouston\tTX\tHarris County\tH1\n77092\t48201\tHouston\tTX\tHarris County\tH1\n77255\t48201\tHouston\tTX\tHarris County\tH1\n77272\t48201\tHouston\tTX\tHarris County\tH1\n77388\t48201\tSpring\tTX\tHarris County\tH1\n77429\t48201\tCypress\tTX\tHarris County\tH1\n77051\t48201\tHouston\tTX\tHarris County\tH1\n77057\t48201\tHouston\tTX\tHarris County\tH1\n77033\t48201\tHouston\tTX\tHarris County\tH1\n77049\t48201\tHouston\tTX\tHarris County\tH1\n77028\t48201\tHouston\tTX\tHarris County\tH1\n77064\t48201\tHouston\tTX\tHarris County\tH1\n77493\t48201\tKaty\tTX\tHarris County\tH1\n77505\t48201\tPasadena\tTX\tHarris County\tH1\n77275\t48201\tHouston\tTX\tHarris County\tH1\n77263\t48201\tHouston\tTX\tHarris County\tH1\n77262\t48201\tHouston\tTX\tHarris County\tH1\n77240\t48201\tHouston\tTX\tHarris County\tH1\n77222\t48201\tHouston\tTX\tHarris County\tH1\n77267\t48201\tHouston\tTX\tHarris County\tH1\n77236\t48201\tHouston\tTX\tHarris County\tH1\n77271\t48201\tHouston\tTX\tHarris County\tH1\n77014\t48201\tHouston\tTX\tHarris County\tH1\n77020\t48201\tHouston\tTX\tHarris County\tH1\n77004\t48201\tHouston\tTX\tHarris County\tH1\n77018\t48201\tHouston\tTX\tHarris County\tH1\n77003\t48201\tHouston\tTX\tHarris County\tH1\n77084\t48201\tHouston\tTX\tHarris County\tH1\n77089\t48201\tHouston\tTX\tHarris County\tH1\n77091\t48201\tHouston\tTX\tHarris County\tH1\n77072\t48201\tHouston\tTX\tHarris County\tH1\n77070\t48201\tHouston\tTX\tHarris County\tH1\n77094\t48201\tHouston\tTX\tHarris County\tH1\n77098\t48201\tHouston\tTX\tHarris County\tH1\n77085\t48201\tHouston\tTX\tHarris County\tH1\n77346\t48201\tHumble\tTX\tHarris County\tH1\n77254\t48201\tHouston\tTX\tHarris County\tH1\n77257\t48201\tHouston\tTX\tHarris County\tH1\n77410\t48201\tCypress\tTX\tHarris County\tH1\n77048\t48201\tHouston\tTX\tHarris County\tH1\n77029\t48201\tHouston\tTX\tHarris County\tH1\n77063\t48201\tHouston\tTX\tHarris County\tH1\n77041\t48201\tHouston\tTX\tHarris County\tH1\n77445\t48201\tHempstead\tTX\tHarris County\tH1\n77532\t48201\tCrosby\tTX\tHarris County\tH1\n77571\t48201\tLa porte\tTX\tHarris County\tH1\n77225\t48201\tHouston\tTX\tHarris County\tH1\n77234\t48201\tHouston\tTX\tHarris County\tH1\n77259\t48201\tHouston\tTX\tHarris County\tH1\n77413\t48201\tBarker\tTX\tHarris County\tH1\n77492\t48201\tKaty\tTX\tHarris County\tH1\n77277\t48201\tHouston\tTX\tHarris County\tH1\n77280\t48201\tHouston\tTX\tHarris County\tH1\n77205\t48201\tHouston\tTX\tHarris County\tH1\n77223\t48201\tHouston\tTX\tHarris County\tH1\n77289\t48201\tHouston\tTX\tHarris County\tH1\n77315\t48201\tNorth houston\tTX\tHarris County\tH1\n77235\t48201\tHouston\tTX\tHarris County\tH1\n77009\t48201\tHouston\tTX\tHarris County\tH1\n77019\t48201\tHouston\tTX\tHarris County\tH1\n77022\t48201\tHouston\tTX\tHarris County\tH1\n77026\t48201\tHouston\tTX\tHarris County\tH1\n77069\t48201\tHouston\tTX\tHarris County\tH1\n77086\t48201\tHouston\tTX\tHarris County\tH1\n77208\t48201\tHouston\tTX\tHarris County\tH1\n77338\t48201\tHumble\tTX\tHarris County\tH1\n77339\t48201\tKingwood\tTX\tHarris County\tH1\n77218\t48201\tHouston\tTX\tHarris County\tH1\n77219\t48201\tHouston\tTX\tHarris County\tH1\n77336\t48201\tHuffman\tTX\tHarris County\tH1\n77258\t48201\tHouston\tTX\tHarris County\tH1\n77396\t48201\tHumble\tTX\tHarris County\tH1\n77379\t48201\tSpring\tTX\tHarris County\tH1\n77402\t48201\tBellaire\tTX\tHarris County\tH1\n77039\t48201\tHouston\tTX\tHarris County\tH1\n77032\t48201\tHouston\tTX\tHarris County\tH1\n77447\t48201\tHockley\tTX\tHarris County\tH1\n77450\t48201\tKaty\tTX\tHarris County\tH1\n77530\t48201\tChannelview\tTX\tHarris County\tH1\n77536\t48201\tDeer park\tTX\tHarris County\tH1\n77581\t48201\tPearland\tTX\tHarris County\tH1\n77010\t48201\tHouston\tTX\tHarris County\tH1\n77268\t48201\tHouston\tTX\tHarris County\tH1\n77274\t48201\tHouston\tTX\tHarris County\tH1\n77224\t48201\tHouston\tTX\tHarris County\tH1\n77293\t48201\tHouston\tTX\tHarris County\tH1\n77269\t48201\tHouston\tTX\tHarris County\tH1\n77237\t48201\tHouston\tTX\tHarris County\tH1\n77001\t48201\tHouston\tTX\tHarris County\tH1\n77220\t48201\tHouston\tTX\tHarris County\tH1\n77016\t48201\tHouston\tTX\tHarris County\tH1\n77005\t48201\tHouston\tTX\tHarris County\tH1\n77025\t48201\tHouston\tTX\tHarris County\tH1\n77067\t48201\tHouston\tTX\tHarris County\tH1\n77357\t48201\tNew caney\tTX\tHarris County\tH1\n77365\t48201\tPorter\tTX\tHarris County\tH1\n77282\t48201\tHouston\tTX\tHarris County\tH1\n77056\t48201\tHouston\tTX\tHarris County\tH1\n77055\t48201\tHouston\tTX\tHarris County\tH1\n77059\t48201\tHouston\tTX\tHarris County\tH1\n77062\t48201\tHouston\tTX\tHarris County\tH1\n77058\t48201\tHouston\tTX\tHarris County\tH1\n77503\t48201\tPasadena\tTX\tHarris County\tH1\n77508\t48201\tPasadena\tTX\tHarris County\tH1\n77522\t48201\tBaytown\tTX\tHarris County\tH1\n77291\t48201\tHouston\tTX\tHarris County\tH1\n77228\t48201\tHouston\tTX\tHarris County\tH1\n77290\t48201\tHouston\tTX\tHarris County\tH1\n77249\t48201\tHouston\tTX\tHarris County\tH1\n77217\t48201\tHouston\tTX\tHarris County\tH1\n77011\t48201\tHouston\tTX\tHarris County\tH1\n77077\t48201\tHouston\tTX\tHarris County\tH1\n77078\t48201\tHouston\tTX\tHarris County\tH1\n77083\t48201\tHouston\tTX\tHarris County\tH1\n77066\t48201\tHouston\tTX\tHarris County\tH1\n77345\t48201\tKingwood\tTX\tHarris County\tH1\n77383\t48201\tSpring\tTX\tHarris County\tH1\n77433\t48201\tCypress\tTX\tHarris County\tH1\n77038\t48201\tHouston\tTX\tHarris County\tH1\n77053\t48201\tHouston\tTX\tHarris County\tH1\n77040\t48201\tHouston\tTX\tHarris County\tH1\n77045\t48201\tHouston\tTX\tHarris County\tH1\n77047\t48201\tHouston\tTX\tHarris County\tH1\n77061\t48201\tHouston\tTX\tHarris County\tH1\n77501\t48201\tPasadena\tTX\tHarris County\tH1\n77587\t48201\tSouth houston\tTX\tHarris County\tH1\n77244\t48201\tHouston\tTX\tHarris County\tH1\n77227\t48201\tHouston\tTX\tHarris County\tH1\n77256\t48201\tHouston\tTX\tHarris County\tH1\n77411\t48201\tAlief\tTX\tHarris County\tH1\n77287\t48201\tHouston\tTX\tHarris County\tH1\n77288\t48201\tHouston\tTX\tHarris County\tH1\n77238\t48201\tHouston\tTX\tHarris County\tH1\n77002\t48201\tHouston\tTX\tHarris County\tH1\n77006\t48201\tHouston\tTX\tHarris County\tH1\n77023\t48201\tHouston\tTX\tHarris County\tH1\n77081\t48201\tHouston\tTX\tHarris County\tH1\n77215\t48201\tHouston\tTX\tHarris County\tH1\n77099\t48201\tHouston\tTX\tHarris County\tH1\n77373\t48201\tSpring\tTX\tHarris County\tH1\n77377\t48201\tTomball\tTX\tHarris County\tH1\n77043\t48201\tHouston\tTX\tHarris County\tH1\n77034\t48201\tHouston\tTX\tHarris County\tH1\n77036\t48201\tHouston\tTX\tHarris County\tH1\n77030\t48201\tHouston\tTX\tHarris County\tH1\n77050\t48201\tHouston\tTX\tHarris County\tH1\n77484\t48201\tWaller\tTX\tHarris County\tH1\n77494\t48201\tKaty\tTX\tHarris County\tH1\n77477\t48201\tStafford\tTX\tHarris County\tH1\n77502\t48201\tPasadena\tTX\tHarris County\tH1\n77562\t48201\tHighlands\tTX\tHarris County\tH1\n77523\t48201\tBaytown\tTX\tHarris County\tH1\n77547\t48201\tGalena park\tTX\tHarris County\tH1\n77507\t48201\tPasadena\tTX\tHarris County\tH1\n77586\t48201\tSeabrook\tTX\tHarris County\tH1\n77598\t48201\tWebster\tTX\tHarris County\tH1\n77207\t48201\tHouston\tTX\tHarris County\tH1\n77221\t48201\tHouston\tTX\tHarris County\tH1\n77251\t48201\tHouston\tTX\tHarris County\tH1\n77248\t48201\tHouston\tTX\tHarris County\tH1\n77292\t48201\tHouston\tTX\tHarris County\tH1\n77391\t48201\tSpring\tTX\tHarris County\tH1\n77052\t48201\tHouston\tTX\tHarris County\tH1\n77572\t48201\tLa porte\tTX\tHarris County\tH1\n75605\t48203\tLongview\tTX\tHarrison County\tH1\n75639\t48203\tDe berry\tTX\tHarrison County\tH1\n75659\t48203\tJonesville\tTX\tHarrison County\tH1\n75661\t48203\tKarnack\tTX\tHarrison County\tH1\n75601\t48203\tLongview\tTX\tHarrison County\tH1\n75602\t48203\tLongview\tTX\tHarrison County\tH1\n75670\t48203\tMarshall\tTX\tHarrison County\tH1\n75672\t48203\tMarshall\tTX\tHarrison County\tH1\n75688\t48203\tScottsville\tTX\tHarrison County\tH1\n75642\t48203\tElysian fields\tTX\tHarrison County\tH1\n75650\t48203\tHallsville\tTX\tHarrison County\tH1\n75671\t48203\tMarshall\tTX\tHarrison County\tH1\n75692\t48203\tWaskom\tTX\tHarrison County\tH1\n75657\t48203\tJefferson\tTX\tHarrison County\tH1\n75683\t48203\tOre city\tTX\tHarrison County\tH1\n75651\t48203\tHarleton\tTX\tHarrison County\tH1\n75640\t48203\tDiana\tTX\tHarrison County\tH1\n75694\t48203\tWoodlawn\tTX\tHarrison County\tH1\n79018\t48205\tChanning\tTX\tHartley County\tH1\n79022\t48205\tDalhart\tTX\tHartley County\tH1\n79044\t48205\tHartley\tTX\tHartley County\tH1\n79521\t48207\tHaskell\tTX\tHaskell County\tH1\n76388\t48207\tWeinert\tTX\tHaskell County\tH1\n79553\t48207\tStamford\tTX\tHaskell County\tH1\n79544\t48207\tRochester\tTX\tHaskell County\tH1\n79547\t48207\tRule\tTX\tHaskell County\tH1\n79503\t48207\tAvoca\tTX\tHaskell County\tH1\n79548\t48207\tRule\tTX\tHaskell County\tH1\n79539\t48207\tO brien\tTX\tHaskell County\tH1\n79533\t48207\tLueders\tTX\tHaskell County\tH1\n78132\t48209\tNew braunfels\tTX\tHays County\tH1\n78738\t48209\tAustin\tTX\tHays County\tH1\n78130\t48209\tNew braunfels\tTX\tHays County\tH1\n78652\t48209\tManchaca\tTX\tHays County\tH1\n78620\t48209\tDripping springs\tTX\tHays County\tH1\n78666\t48209\tSan marcos\tTX\tHays County\tH1\n78736\t48209\tAustin\tTX\tHays County\tH1\n78640\t48209\tKyle\tTX\tHays County\tH1\n78610\t48209\tBuda\tTX\tHays County\tH1\n78656\t48209\tMaxwell\tTX\tHays County\tH1\n78623\t48209\tFischer\tTX\tHays County\tH1\n78663\t48209\tRound mountain\tTX\tHays County\tH1\n78619\t48209\tDriftwood\tTX\tHays County\tH1\n78676\t48209\tWimberley\tTX\tHays County\tH1\n78739\t48209\tAustin\tTX\tHays County\tH1\n78737\t48209\tAustin\tTX\tHays County\tH1\n78667\t48209\tSan marcos\tTX\tHays County\tH1\n78606\t48209\tBlanco\tTX\tHays County\tH1\n79014\t48211\tCanadian\tTX\tHemphill County\tH1\n79011\t48211\tBriscoe\tTX\tHemphill County\tH1\n75803\t
